vi "index to z.vi"(7 "number of points":i32, 9 "complex region":T1, 10 "im index":i32, 11 "re index":i32) -> (3 "z":cdb)   [LabVIEW 2010]
uses:
  complex region.ctl
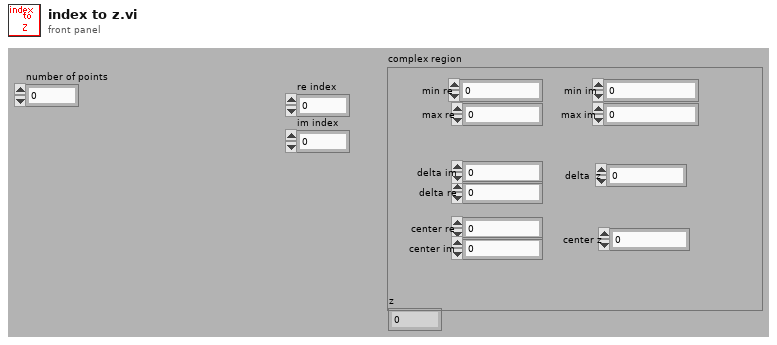
[diagram p1: front panel]
types:
  T1 = typedef "complex region.ctl" = cluster{"max re":dbl, "min re":dbl, "max im":dbl, "min im":dbl, "delta re":dbl, "delta im":dbl, "center re":dbl, "delta  z":cdb, "center im":dbl, "center z":cdb}
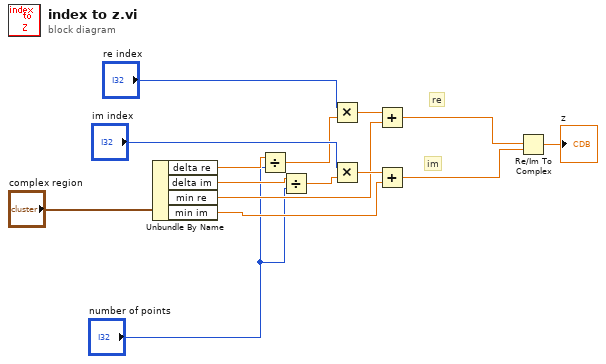
[diagram p0: block diagram]
diagram:
  # "re"
  # "im"
  n1 = Unbundle By Name("complex region") -> ("delta re"=w5:dbl, "delta im"=w3:dbl, "min re"=w11:dbl, "min im"=w9:dbl)
  n2 = Divide(x=w5, y="number of points") -> (x/y=w4:dbl)
  n3 = Divide(x=w3, y="number of points") -> (x/y=w1:dbl)
  n4 = Multiply(x="re index", y=w4) -> (x*y=w15:dbl)
  n5 = Multiply(x="im index", y=w1) -> (x*y=w14:dbl)
  n6 = Add(x=w15, y=w11) -> (x+y=w8:dbl)
  n7 = Add(x=w14, y=w9) -> (x+y=w7:dbl)
  n8 = Re/Im To Complex(1:w7, 2:w8) -> (0:→"z":cdb)
